vi "WriteControlKey.vi"(9 "ConfigFile":T1, 10 "section":string, 11 "Control in":refnum<vi>) -> (3 "ConfigFile out":T1)   [LabVIEW 2016]
uses:
  <vilib>/Utility/config.llb/Config Data RefNum.ctl
  <vilib>/Utility/Data Type/Type Definitions/Data Type.ctl
  <vilib>/Utility/config.llb/Write Key (Path).vi
  <vilib>/Utility/config.llb/Write Key (String).vi
  <vilib>/Utility/config.llb/Write Key (Boolean).vi
  <vilib>/Utility/config.llb/Write Key (Double).vi
  <vilib>/Utility/config.llb/Write Key (I32).vi
  <vilib>/Utility/Data Type/NI_Data Type.lvlib
  <vilib>/Utility/config.llb/NI_LVConfig.lvlib
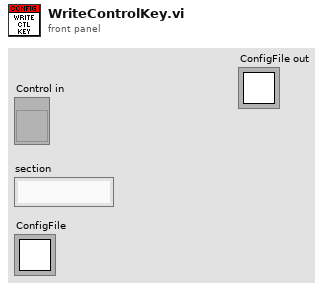
[diagram p1: front panel]
types:
  T1 = typedef "NI_LVConfig.lvlib/Config Data RefNum.ctl" = refnum<k1>
  T2 = typedef "NI_Data Type.lvlib/Data Type.ctl" = enum8{"Invalid Type", "Void", "I8", "I16", "I32", "I64", "U8", "U16", "U32", "U64", "Single Float", "Double Float", "Extended Float", "Single Complex", "Double Complex", "Extended Complex", "Enum U8", "Enum U16", "Enum U32", "Enum U64", "Single Float With Unit", "Double Float With Unit", "Extended Float With Unit", "Single Complex with Unit", "Double Complex with Unit", "Extended Complex with Unit", "Boolean", "String", "Path", "Picture", "Tag", "Array", "Cluster", "Variant", "LV Variant", "Waveform", "Timestamp", "Digital Waveform", "Digital Data", "ExpressData", "Refnum", "External Data", "VI", "Poly VI", "LabVIEW Class Instance", "Fixed Point"}
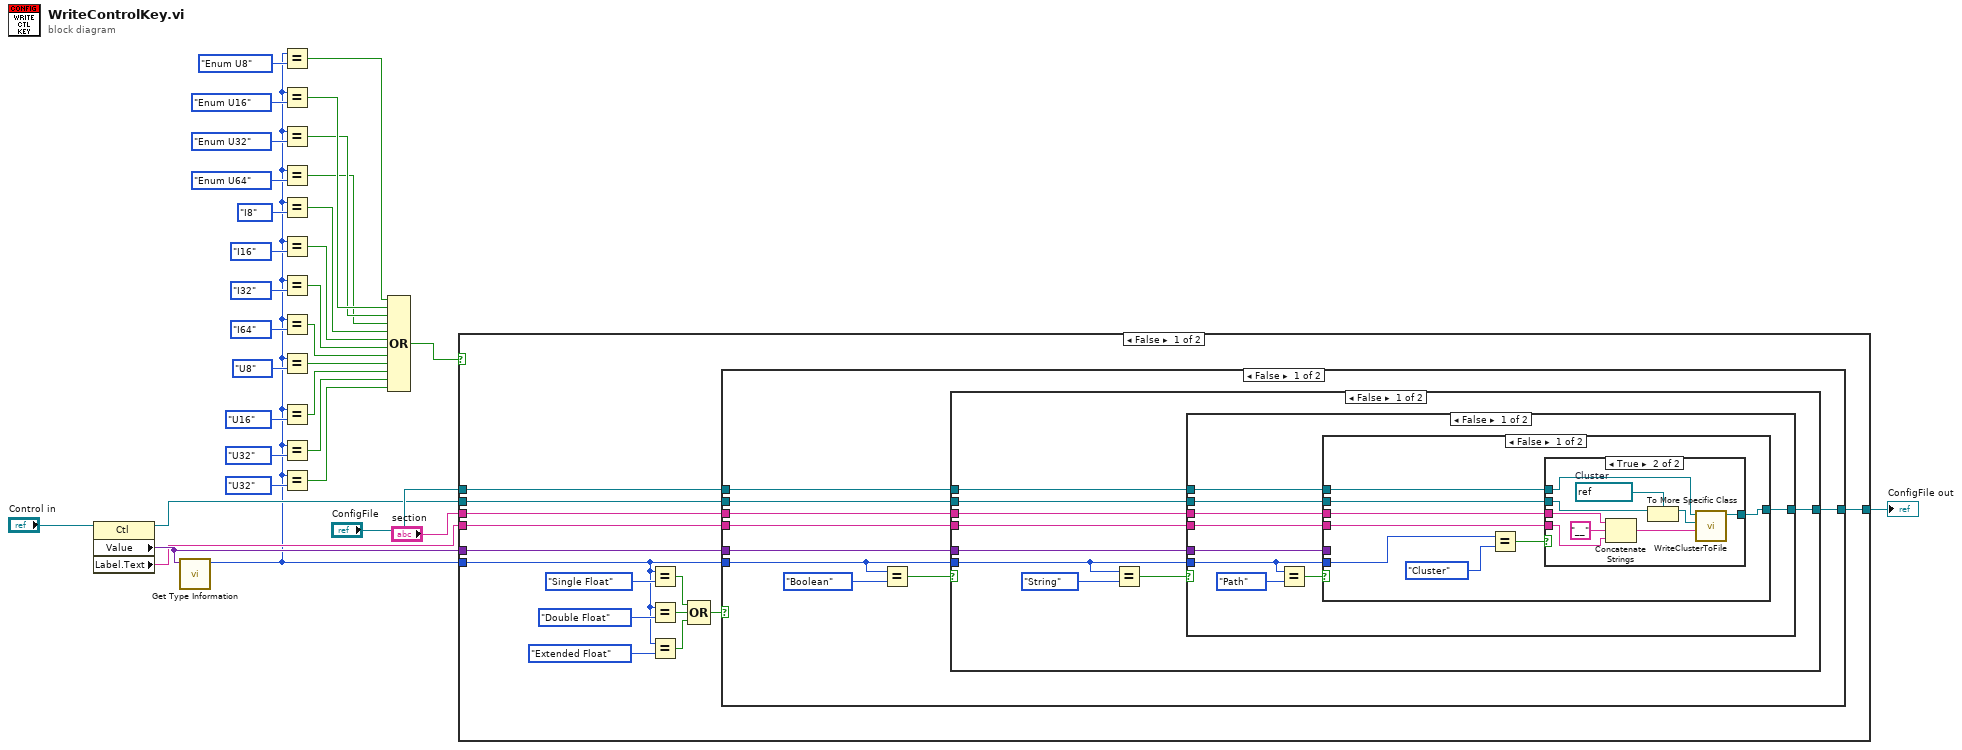
[diagram p0: block diagram]
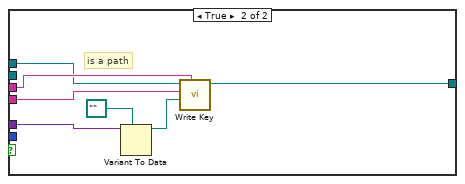
[diagram p3: hidden frame]
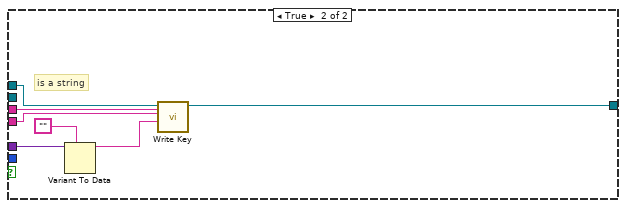
[diagram p4: hidden frame]
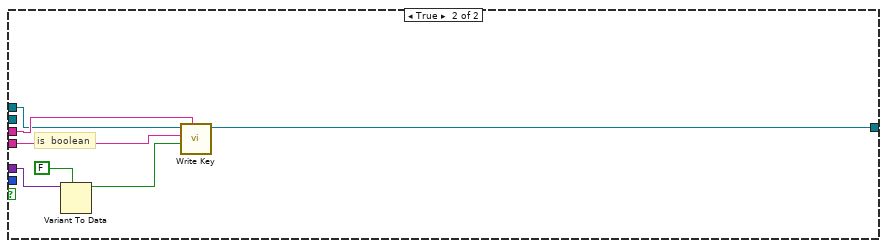
[diagram p5: hidden frame]
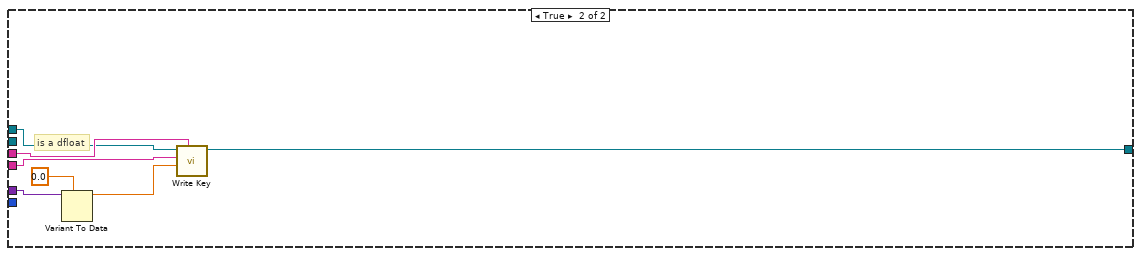
[diagram p6: hidden frame]
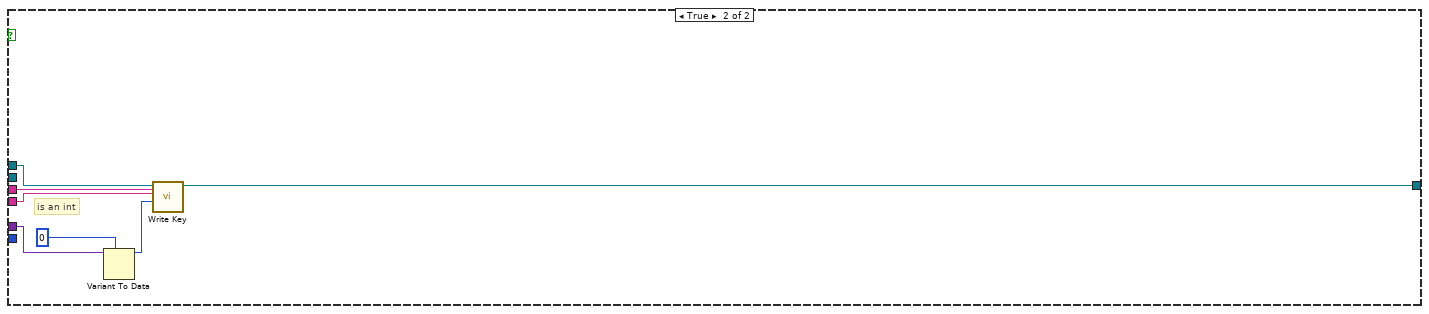
[diagram p7: hidden frame]
diagram:
  n1 = property class="Ctl"(reference="Control in") -> (reference out=w11:refnum<vi>, "Value"=w31:variant, "Label.Text"=w10:string)  [unwired: 1 in, 1 out]
  n2 = call <vilib>:"Get Type Information.vi"("Variant"=w31) -> ("Type"=w5:T2)  [unwired: 6 in, 4 out]
  n3 = Equal?(x=w5, y=Data_Type."Enum U8" ("Type")) -> (x = y?=w4:bool)
  n4 = Equal?(x=w5, y=Data_Type."Enum U16" ("Type")) -> (x = y?=w3:bool)
  n5 = Equal?(x=w5, y=Data_Type."Enum U32" ("Type")) -> (x = y?=w2:bool)
  n6 = Equal?(x=w5, y=Data_Type."Enum U64" ("Type")) -> (x = y?=w1:bool)
  n7 = Equal?(x=w5, y=Data_Type."I8" ("Type")) -> (x = y?=w22:bool)
  n8 = Equal?(x=w5, y=Data_Type."I16" ("Type")) -> (x = y?=w23:bool)
  n9 = Equal?(x=w5, y=Data_Type."I32" ("Type")) -> (x = y?=w24:bool)
  n10 = Equal?(x=w5, y=Data_Type."I64" ("Type")) -> (x = y?=w25:bool)
  n11 = Equal?(x=w5, y=Data_Type."U8" ("Type")) -> (x = y?=w26:bool)
  n12 = Equal?(x=w5, y=Data_Type."U16" ("Type")) -> (x = y?=w27:bool)
  n13 = Equal?(x=w5, y=Data_Type."U32" ("Type")) -> (x = y?=w28:bool)
  n14 = Equal?(x=w5, y=Data_Type."U32" ("Type")) -> (x = y?=w29:bool)
  n15 = Compound Arithmetic op=OR(w4, w3, w2, w1, w22, w23, w24, w25, w26, w27, w28, w29) -> (w30:bool)
  n16 = case shown="False" w30 {
    tunnel: w5 -> [w40 _]
    tunnel: w31 -> [w39 w126]
    tunnel: w10 -> [w38 w123]
    tunnel: "ConfigFile" -> [w36 w127]
    tunnel: "section" -> [w37 w122]
    tunnel: [w35 w121] -> w12
    tunnel: w11 -> [w34 _]
    frame False {
      n17 = Equal?(x=w40, y=Data_Type."Single Float" ("Type")) -> (x = y?=w44:bool)
      n18 = Equal?(x=w40, y=Data_Type."Double Float" ("Type")) -> (x = y?=w43:bool)
      n19 = Equal?(x=w40, y=Data_Type."Extended Float" ("Type")) -> (x = y?=w42:bool)
      n20 = Compound Arithmetic op=OR(w44, w43, w42) -> (w41:bool)
      n21 = case shown="False" w41 {
        tunnel: w40 -> [w54 _]
        tunnel: w39 -> [w53 w116]
        tunnel: w38 -> [w52 w117]
        tunnel: w37 -> [w51 w118]
        tunnel: w36 -> [w50 w115]
        tunnel: [w49 w114] -> w35
        tunnel: w34 -> [w48 _]
        frame False {
          n22 = Equal?(x=w54, y=Data_Type."Boolean" ("Type")) -> (x = y?=w55:bool)
          n23 = case shown="False" w55 {
            tunnel: w54 -> [w63 _]
            tunnel: w53 -> [w62 w108]
            tunnel: w52 -> [w61 w109]
            tunnel: w51 -> [w60 w111]
            tunnel: w50 -> [w59 w110]
            tunnel: [w58 w107] -> w49
            tunnel: w48 -> [w57 _]
            frame False {
              n24 = Equal?(x=w63, y=Data_Type."String" ("Type")) -> (x = y?=w64:bool)
              n25 = case shown="False" w64 {
                tunnel: w63 -> [w67 _]
                tunnel: w62 -> [w72 w101]
                tunnel: w61 -> [w71 w102]
                tunnel: w60 -> [w70 w104]
                tunnel: w59 -> [w69 w103]
                tunnel: [w68 w100] -> w58
                tunnel: w57 -> [w66 _]
                frame False {
                  n26 = Equal?(x=w67, y=Data_Type."Path" ("Type")) -> (x = y?=w73:bool)
                  n27 = case shown="False" w73 {
                    tunnel: w72 -> [_ w94]
                    tunnel: w71 -> [w75 w95]
                    tunnel: w70 -> [w77 w97]
                    tunnel: w69 -> [w79 w96]
                    tunnel: [w76 w93] -> w68
                    tunnel: w67 -> [w82 _]
                    tunnel: w66 -> [w78 _]
                    frame False {
                      n28 = Equal?(x=w82, y=Data_Type."Cluster") -> (x = y?=w80:bool)
                      n29 = case shown="True" w80 {
                        tunnel: w79 -> [w83 w92]
                        tunnel: w78 -> [_ w91]
                        tunnel: w77 -> [_ w88]
                        tunnel: [w83 w85] -> w76
                        tunnel: w75 -> [_ w84]
                        frame False {
                        }
                        frame True {
                          w90 = refnum<vi> refnum  # Cluster
                          n30 = Concatenate Strings(w88, "__" ("string"), w84) -> (w86:string)
                          n31 = To More Specific Class(target class=w90, reference=w91) -> (specific class reference=w89:refnum<vi>)  [unwired: 1 in, 1 out]
                          n32 = call "WriteClusterToFile.vi"("Name"=w86, "Cluster in"=w89, "ConfigIn"=w92) -> ("ConfigOut"=w85:T1)  [unwired: 8 in]
                        }
                      }
                    }
                    frame True {
                      # "is a path"
                      n33 = Variant To Data(type=path "", Variant=w94) -> (data=w98:path)  [unwired: 1 in, 1 out]
                      n34 = call-poly <vilib>:"Write Key.vi"("section"=w97, "value"=w98, "key"=w95, "refnum"=w96) -> ("refnum out"=w93:T1)  [unwired: 5 in, 2 out]
                    }
                  }
                }
                frame True {
                  # "is a string"
                  n35 = Variant To Data(type="", Variant=w101) -> (data=w105:string)  [unwired: 1 in, 1 out]
                  n36 = call-poly <vilib>:"Write Key.vi"("section"=w104, "value"=w105, "key"=w102, "refnum"=w103) -> ("refnum out"=w100:T1)  [unwired: 5 in, 2 out]
                }
              }
            }
            frame True {
              # "is  boolean"
              n37 = Variant To Data(type=FALSE, Variant=w108) -> (data=w112:bool)  [unwired: 1 in, 1 out]
              n38 = call-poly <vilib>:"Write Key.vi"("section"=w111, "value"=w112, "key"=w109, "refnum"=w110) -> ("refnum out"=w107:T1)  [unwired: 5 in, 2 out]
            }
          }
        }
        frame True {
          # "is a dfloat"
          n39 = Variant To Data(type=0.0, Variant=w116) -> (data=w119:dbl)  [unwired: 1 in, 1 out]
          n40 = call-poly <vilib>:"Write Key.vi"("section"=w118, "value"=w119, "key"=w117, "refnum"=w115) -> ("refnum out"=w114:T1)  [unwired: 5 in, 2 out]
        }
      }
    }
    frame True {
      # "is an int"
      n41 = Variant To Data(type=0, Variant=w126) -> (data=w124:i32)  [unwired: 1 in, 1 out]
      n42 = call-poly <vilib>:"Write Key.vi"("section"=w122, "value"=w124, "key"=w123, "refnum"=w127) -> ("refnum out"=w121:T1)  [unwired: 5 in, 2 out]
    }
  }
  "ConfigFile out" <- w12
